vi "Request Handlers.vi"(4 "WebSocket Handler":refnum<class "WebSocket Handler.lvclass">, 6 "WebSocket Handling":bool, 9 "Request Handler Map":T1, 11 "Processing In":refnum<class "Processing.lvclass">) -> (0 "error out":errorcluster, 2 "Early Response?":bool, 3 "HTTP Server.lvlib:Processing":refnum<class "Processing.lvclass">)   [LabVIEW 2020, in "HTTP Server.lvlib" / "Server.lvclass"]
uses:
  Server.lvclass
  Server.lvclass/Server.ctl
  Processing/Processing.lvclass
  Processing Step.ctl
  HTTP Server.lvlib
  HTTPS Redirect Handler/HTTPS Redirect Handler.lvclass
  Request Handler/Request Handler.lvclass
  WebSocket Handler/WebSocket Handler.lvclass
  C:/dev/lv20CE/relink/lv-http-server/HTTP Server/Complete Handler/Complete Handler.lvclass
  C:/dev/lv20CE/relink/lv-http-server/HTTP Server/Handler/Handler.lvclass
  C:/dev/lv20CE/relink/lv-http-server/HTTP Server/Exception Handler/Exception Handler.lvclass
  C:/dev/lv20CE/relink/lv-http-server/HTTP Server/Request Handler/Request Handler.lvclass
  C:/dev/lv20CE/relink/lv-http-server/HTTP Server/Response Handler/Response Handler.lvclass
  C:/dev/lv20CE/relink/lv-http-server/HTTP Server/WebSocket Handler/WebSocket Handler.lvclass
  Priority.ctl
  Request Handler Map.ctl
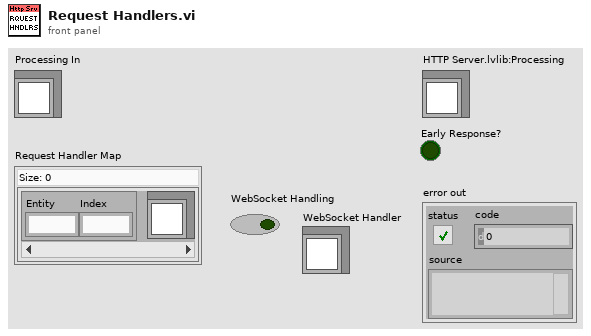
[diagram p1: front panel]
types:
  T1 = typedef "HTTP Server.lvlib/Request Handler Map.ctl" = map{T2, refnum<class "Request Handler.lvclass">}
  T2 = typedef "HTTP Server.lvlib/Priority.ctl" = cluster{"Entity":u16, "Index":u16}
  T3 = typedef "HTTP Server.lvlib/Processing Step.ctl" = enum16{"Connection", "Request", "Routing", "Controller Init", "Controller", "Response", "Complete", "Exception"}
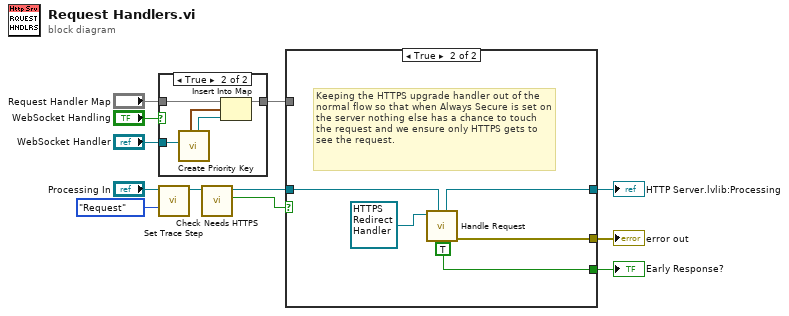
[diagram p0: block diagram]
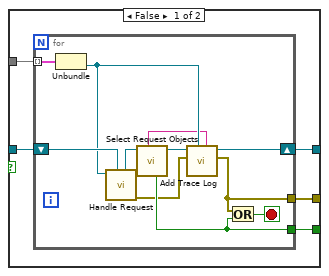
[diagram p3: hidden frame]
diagram:
  n1 = case shown="True" "WebSocket Handling" {
    tunnel: "Request Handler Map" -> [w13 w16]
    tunnel: "WebSocket Handler" -> [_ w14]
    tunnel: [w13 w15] -> w7
    frame False {
    }
    frame True {
      n2 = call "Create Priority Key.vi"("Handler In"=w14) -> ("Handler"=w17:refnum<class "WebSocket Handler.lvclass">, "Priority Key"=w18:T2)  [unwired: 8 in, 1 out]
      n3 = Insert Into Map(map in=w16, key=w18, value=w17) -> (map out=w15:T1)  [unwired: 2 out]
    }
  }
  n4 = call "Set Trace Step.vi"("Processing Step"=Processing_Step."Request", "Processing in"="Processing In") -> ("Processing out"=w3:refnum<class "Processing.lvclass">)  [unwired: 9 in]
  n5 = call "Check Needs HTTPS.vi"("Processing In"=w3) -> ("HTTPS Upgrade?"=w1:bool, "Processing out"=w2:refnum<class "Processing.lvclass">)  [unwired: 8 in, 1 out]
  n6 = case shown="True" w1 {
    tunnel: [w23 w37] -> w11
    tunnel: [w22 TRUE ("Early Response?")] -> w10
    tunnel: w7 -> [w21 _]
    tunnel: [w20 w38] -> w5
    tunnel: w2 -> [w19 w39]
    frame False {
      n7 = for {
        tunnel: w21 -> [w34] mode=indexing
        tunnel: [w25] -> w23
        shift-right: [w24] -> w20
        shift-left: w19 -> [w32]
        tunnel: [w31] -> w22
        stop <- w33 stop-if-true
        n8 = Unbundle(w34) -> ("Handler"=w28:refnum<class "Request Handler.lvclass">)  [unwired: 1 out]
        n9 = call-dynamic "Handle Request.vi"("Processing In"=w32, "Request Handler in"=w28) -> ("error out"=w26:errorcluster, "Processing"=w30:refnum<class "Processing.lvclass">)  [unwired: 8 in]
        n10 = call "Select Request Objects.vi"("Processing In"=w30) -> ("Processing"=w29:refnum<class "Processing.lvclass">, "Early Response?"=w31:bool, "Trace Message"=w27:string)  [unwired: 8 in]
        n11 = call "Add Trace Log.vi"("Info"=w27, "LabVIEW Object"=w28, "error in (no error)"=w26, "Processing in"=w29) -> ("error out"=w25:errorcluster, "Processing out"=w24:refnum<class "Processing.lvclass">)  [unwired: 6 in]
        n12 = Or(x=w25, y=w31) -> (x .or. y?=w33:bool)
      }
    }
    frame True {
      # "Keeping the HTTPS upgrade handler out of the normal flow so that when Always Secure is set on the server nothing else has a chance to touch the request and we ensure only HTTPS gets to see the request."
      n13 = call-dynamic "Handle Request.vi"("Processing In"=w39, "HTTPS Redirect Handler in"=refnum<class "HTTPS Redirect Handler.lvclass"> refnum) -> ("error out"=w37:errorcluster, "Processing"=w38:refnum<class "Processing.lvclass">)  [unwired: 8 in]
    }
  }
  "HTTP Server.lvlib:Processing" <- w5
  "error out" <- w11
  "Early Response?" <- w10
